vi "Folder - Create Application Folders.vi"(10 "ControlsOnPage":refnum<vi>[](array[refnum]), 11 "SRTRS4070 Folder":string) -> (0 "error out":errorcluster, 3 "Paths":path[](array[path]))   [LabVIEW 2013]
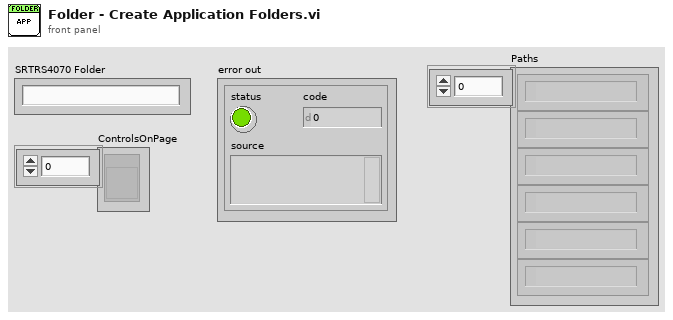
[diagram p1: front panel]
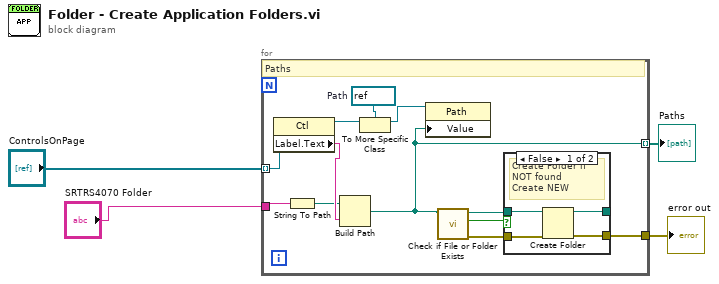
[diagram p0: block diagram]
diagram:
  n1 = for {
    tunnel: "SRTRS4070 Folder" -> [w16]
    tunnel: "ControlsOnPage" -> [w15] mode=indexing
    tunnel: [w7] -> w2
    tunnel: [w5] -> w1 mode=indexing
    w13 = refnum<vi> refnum  # Path
    # "Paths"
    n2 = property class="Ctl"(reference=w15) -> (reference out=w12:refnum<vi>, "Label.Text"=w14:string)  [unwired: 1 in, 1 out]
    n3 = String To Path(string=w16) -> (path=w6:path)
    n4 = Build Path(base path=w6, name or relative path=w14) -> (appended path=w5:path)
    n5 = To More Specific Class(target class=w13, reference=w12) -> (specific class reference=w11:refnum<vi>)  [unwired: 1 in, 1 out]
    n6 = property class="Path"(reference=w11, "Value"=w5) -> ()  [unwired: 1 in, 2 out]
    n7 = call <vilib>:"Check if File or Folder Exists.vi"("path"=w5) -> ("error out"=w8:errorcluster, "file or folder exists?"=w10:bool, "dup path"=w9:path)  [unwired: 8 in]
    n8 = case shown="False" w10 {
      tunnel: w9 -> [w20 w22]
      tunnel: [w19 w22] -> _
      tunnel: [w18 w21] -> w7
      tunnel: w8 -> [w17 w21]
      frame False {
        # "Create Folder if NOT found\nCreate NEW"
        n9 = Create Folder(path (use dialog)=w20, error in=w17) -> (created path=w19:path, error out=w18:errorcluster)  [unwired: 1 in, 1 out]
      }
      frame True {
        # "Folder Found"
      }
    }
  }
  "error out" <- w2
  "Paths" <- w1
